vi "Inst.Transport.CallByReference.vi"(8 "error in (no error)":errorcluster, 9 "VI":T1=enum."LockinTimeDelay", 10 "vi path":path, 11 "Transport":refnum<class "Transport.lvclass">) -> (0 "error out":errorcluster)   [LabVIEW 2019, in "Inst.Transport.lvclass"]
uses:
  Inst.Transport.lvclass
  Transport/Transport.lvclass
  Typedefs/Inst.Transport.Methods--Enum.ctl
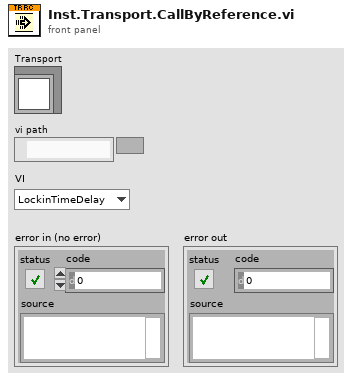
[diagram p1: front panel]
types:
  T1 = typedef "Inst.Transport.lvclass/Inst.Transport.Methods--Enum.ctl" = enum16{"LockinSweep", "LockinTime", "LockinTimeDelay"}
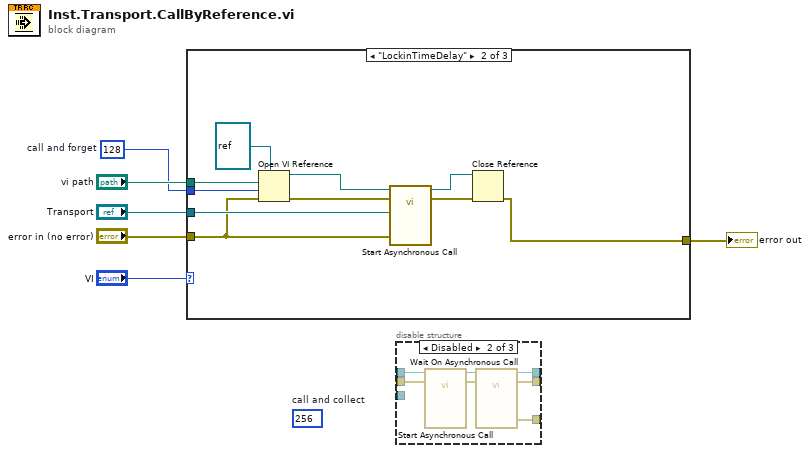
[diagram p0: block diagram]
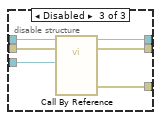
[diagram p3: hidden frame]
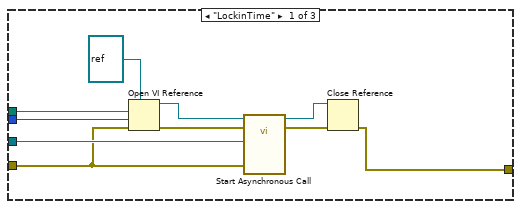
[diagram p4: hidden frame]
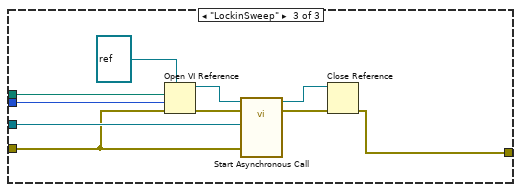
[diagram p5: hidden frame]
diagram:
  (unwired) 256  # call and collect
  w1 = 128  # call and forget
  n1 = case shown="\"LockinTimeDelay\"" "VI" {
    tunnel: "vi path" -> [w14 w24 w36]
    tunnel: "Transport" -> [w12 w22 w35]
    tunnel: [w9 w19 w31] -> w2
    tunnel: "error in (no error)" -> [w8 w18 w28]
    tunnel: w1 -> [w7 w17 w27]
    frame "LockinTime" {
      n2 = Open VI Reference(type specifier VI Refnum (for type only)=refnum<vi> refnum, vi path=w14, options=w7, error in (no error)=w8) -> (vi reference=w13:refnum<vi>, error out=w15:errorcluster)  [unwired: 2 in]
      n3 = call-by-ref "Start Asynchronous Call"(reference=w13, error in=w15, 8:"error in (no error)"=w8, "Transport"=w12) -> (reference out=w10:refnum<vi>, error out=w11:errorcluster)  [unwired: 8 in, 2 out]
      n4 = Close Reference(reference=w10, error in (no error)=w11) -> (error out=w9:errorcluster)
    }
    frame "LockinTimeDelay" {
      n5 = Open VI Reference(type specifier VI Refnum (for type only)=refnum<vi> refnum, vi path=w24, options=w17, error in (no error)=w18) -> (vi reference=w23:refnum<vi>, error out=w25:errorcluster)  [unwired: 2 in]
      n6 = call-by-ref "Start Asynchronous Call"(reference=w23, error in=w25, 8:"error in (no error)"=w18, "Transport"=w22) -> (reference out=w21:refnum<vi>, error out=w20:errorcluster)  [unwired: 8 in, 2 out]
      n7 = Close Reference(reference=w21, error in (no error)=w20) -> (error out=w19:errorcluster)
    }
    frame "LockinSweep" {
      n8 = Open VI Reference(type specifier VI Refnum (for type only)=refnum<vi> refnum, vi path=w36, options=w27, error in (no error)=w28) -> (vi reference=w34:refnum<vi>, error out=w30:errorcluster)  [unwired: 2 in]
      n9 = call-by-ref "Start Asynchronous Call"(reference=w34, error in=w30, "Transport"=w35, 3:"error in (no error)"=w28) -> (reference out=w32:refnum<vi>, error out=w29:errorcluster)  [unwired: 7 in, 2 out]
      n10 = Close Reference(reference=w32, error in (no error)=w29) -> (error out=w31:errorcluster)
    }
  }
  "error out" <- w2
  n11 = disable-structure shown="Disabled" {
    disable-tunnel: _ -> [_ w43 w46]
    disable-tunnel: [_ w40 w47] -> _
    disable-tunnel: _ -> [_ w39 w49]
    disable-tunnel: [_ w38 w48] -> _
    disable-tunnel: _ -> [_ _ w45]
    disable-tunnel: [_ w37 w44] -> _
    frame Enabled {
    }
    frame Disabled {
      n12 = call-by-ref "Start Asynchronous Call"(reference=w39, error in=w43) -> (reference out=w42:refnum<vi>, error out=w41:errorcluster)  [unwired: 10 in, 2 out]
      n13 = call-by-ref "Wait On Asynchronous Call"(reference=w42, error in=w41) -> (reference out=w38:refnum<vi>, error out=w40:errorcluster, 0:"error out"=w37:errorcluster)  [unwired: 10 in, 1 out]
    }
    frame Disabled {
      n14 = call-by-ref "?"(reference=w49, error in=w46, "Transport"=w45) -> (reference out=w48:refnum<vi>, error out=w47:errorcluster, 0:"error out"=w44:errorcluster)  [unwired: 9 in, 1 out]
    }
  }
